vi "Create.vi"(5 "CF (kHz)":dbl=8.0 format="%#_13g", 9 "BW (kHz)":dbl=0.5 format="%#_13g") -> (8 "Filter":refnum<class "Filter.lvclass">)   [LabVIEW 2020, in "Filter.lvclass"]
uses:
  Filter.lvclass
  Shape.ctl
  Units.ctl
  Class.ctl
  Filter.lvclass/Filter.ctl
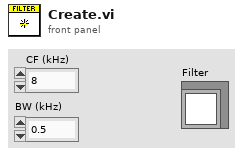
[diagram p1: front panel]
types:
  T1 = typedef "Filter.lvclass/Class.ctl" = enum16{"Elliptic", "Butterworth", "Brickwall"}
  T2 = typedef "Filter.lvclass/Units.ctl" = enum16{"Linear", "Octaves", "Min-Max"}
  T3 = typedef "Filter.lvclass/Shape.ctl" = enum16{"OFF", "Lowpass", "Highpass", "Bandpass", "Bandstop"}
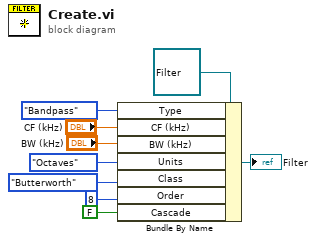
[diagram p0: block diagram]
diagram:
  n1 = Bundle By Name(cluster=refnum<class "Filter.lvclass"> refnum ("Filter"), "Type"=Shape."Bandpass" ("Serialized.Type"), "CF (kHz)"="CF (kHz)", "BW (kHz)"="BW (kHz)", "Units"=Units."Octaves" ("Serialized.Units"), "Class"=Class."Butterworth" ("Serialized.Class"), "Order"=8 ("Serialized.Order"), "Cascade"=FALSE ("Serialized.Cascade")) -> (→"Filter":refnum<class "Filter.lvclass">)
